vi "Command Distance RPED Right.vi"(8 "Timeout":u32, 10 "Distance":dbl format="%#_13g", 11 "Startup":bool) -> (2 "RPED Right":dbl, 4 "Reinit":bool, 5 "Completed":bool)   [LabVIEW 2017]
uses:
  Drive/Drive Globals.vi
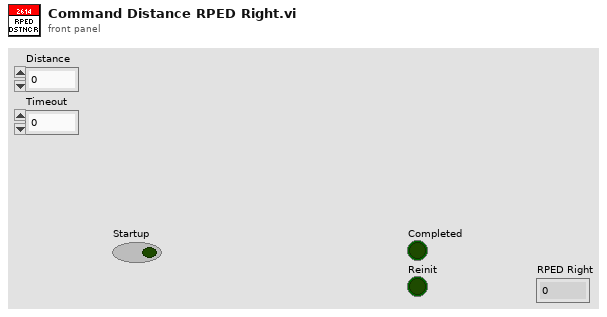
[diagram p1: front panel]
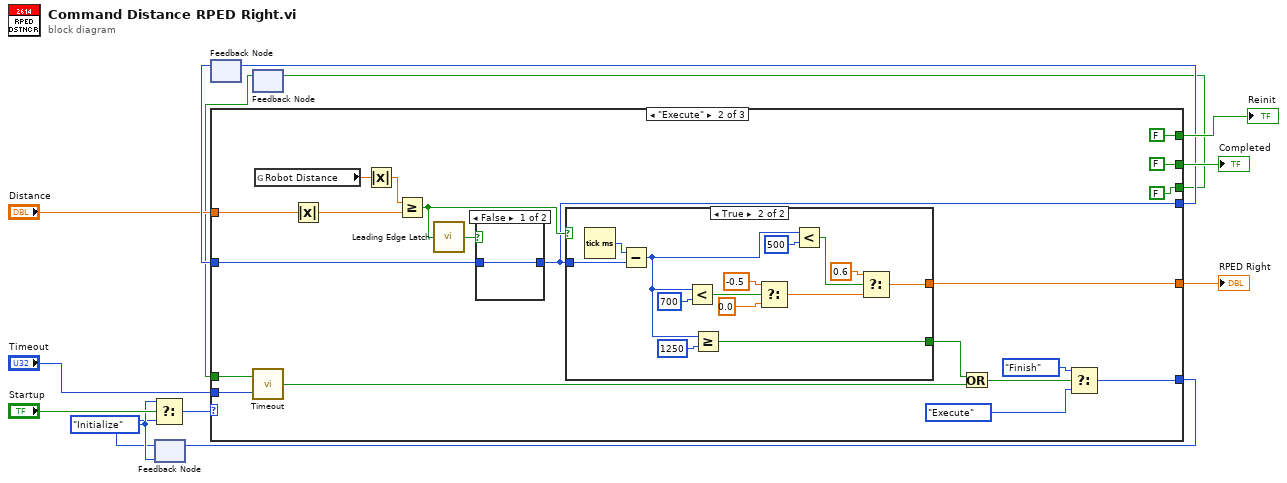
[diagram p0: block diagram]
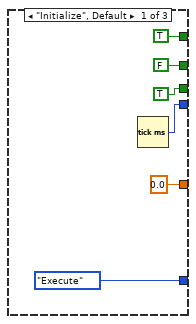
[diagram p2: hidden frame]
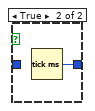
[diagram p3: hidden frame]
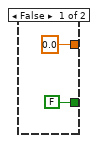
[diagram p4: hidden frame]
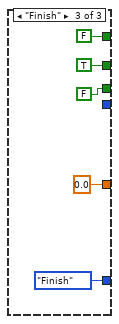
[diagram p5: hidden frame]
diagram:
  w12 = enum16{"Initialize", "Execute", "Finish"}."Initialize"
  n1 = feedback #1(w12) -> (w7:enum16{"Initialize", "Execute", "Finish"})
  n2 = Select(t=w12, s="Startup", f=w7) -> (s? t:f=w13:enum16{"Initialize", "Execute", "Finish"})
  n3 = feedback #2() -> (w6:u32)  [unwired: 1 in]
  n4 = feedback #3() -> (w2:bool)  [unwired: 1 in]
  n5 = case shown="\"Execute\"" w13 {
    tunnel: [FALSE FALSE TRUE] -> w11
    tunnel: [TRUE FALSE FALSE] -> w10
    tunnel: [enum16{"Initialize", "Execute", "Finish"}."Execute" w34 enum16{"Initialize", "Execute", "Finish"}."Finish"] -> w9
    tunnel: [w17 w21 _] -> w8
    tunnel: w6 -> [_ w22 _]
    tunnel: [0.0 ("Left Wheel Velocity") w38 0.0] -> w5
    tunnel: "Distance" -> [_ w28 _]
    tunnel: [TRUE FALSE FALSE] -> w3
    tunnel: w2 -> [_ w31 _]
    tunnel: "Timeout" -> [_ w30 _]
    frame "Initialize", Default {
      n6 = Tick Count (ms)() -> (millisecond timer value=w17:u32)
    }
    frame "Execute" {
      n7 = call "Timeout.vi"("Timeout"=w30, "Initialize"=w31) -> ("Timed Out?"=w32:bool)
      n8 = global read "Drive Globals.vi" "Robot Distance"() -> (w27:dbl)
      n9 = Absolute Value(x=w28) -> (abs(x)=w26:dbl)
      n10 = Absolute Value(x=w27) -> (abs(x)=w25:dbl)
      n11 = Greater Or Equal?(x=w25, y=w26) -> (x >= y?=w23:bool)
      n12 = call "Leading Edge Latch.vi"("Input"=w23) -> ("Output"=w24:bool)
      n13 = case shown="False" w24 {
        tunnel: [w41 w42] -> w21
        tunnel: w22 -> [w41 _]
        frame False {
        }
        frame True {
          n14 = Tick Count (ms)() -> (millisecond timer value=w42:u32)
        }
      }
      n15 = case shown="True" w23 {
        tunnel: w21 -> [_ w57]
        tunnel: [0.0 w54] -> w38
        tunnel: [FALSE w45] -> w35
        frame False {
        }
        frame True {
          n16 = Tick Count (ms)() -> (millisecond timer value=w58:u32)
          n17 = Subtract(x=w58, y=w57) -> (x-y=w47:u32)
          n18 = Less?(x=w47, y=u32 700) -> (x < y?=w51:bool)
          n19 = Greater Or Equal?(x=w47, y=u32 1250) -> (x >= y?=w45:bool)
          n20 = Select(t=-0.5, s=w51, f=0.0) -> (s? t:f=w52:dbl)
          n21 = Less?(x=w47, y=u32 500) -> (x < y?=w55:bool)
          n22 = Select(t=0.6, s=w55, f=w52) -> (s? t:f=w54:dbl)
        }
      }
      n23 = Or(x=w35, y=w32) -> (x .or. y?=w33:bool)
      n24 = Select(t=enum16{"Initialize", "Execute", "Finish"}."Finish", s=w33, f=enum16{"Initialize", "Execute", "Finish"}."Execute") -> (s? t:f=w34:enum16{"Initialize", "Execute", "Finish"})
    }
    frame "Finish" {
    }
  }
  "Completed" <- w11
  "Reinit" <- w10
  "RPED Right" <- w5
  n25 = feedback-in #1(w9) -> ()
  n26 = feedback-in #2(w8) -> ()
  n27 = feedback-in #3(w3) -> ()
